vi "SFOAE-Dispose Of Datafile.vi"(0 "Notes":string, 1 "Expt State in":T2, 7 "DataProc":T1, 11 "error in (no error)":errorcluster, 12 "abort":bool) -> (3 "Expt State out":T2, 4 "DataPath":path, 15 "error out":errorcluster)   [LabVIEW 2020]
uses:
  CFTS Main Panel SubVIs/CFTS-Experiment State.ctl
  Typedefs/SFOAE-Data Processing.ctl
  CFTS Main Panel SubVIs/CFTS-Data Type Enum.ctl
  epl-vi-lib/Utility VIs/Math VIs/LinSpace (x0-dx-npts).vi
  epl-vi-lib/Utility VIs/Math VIs/Linear to dB (2D).vi
  <vilib>/regexp/Match Regular Expression.xnode
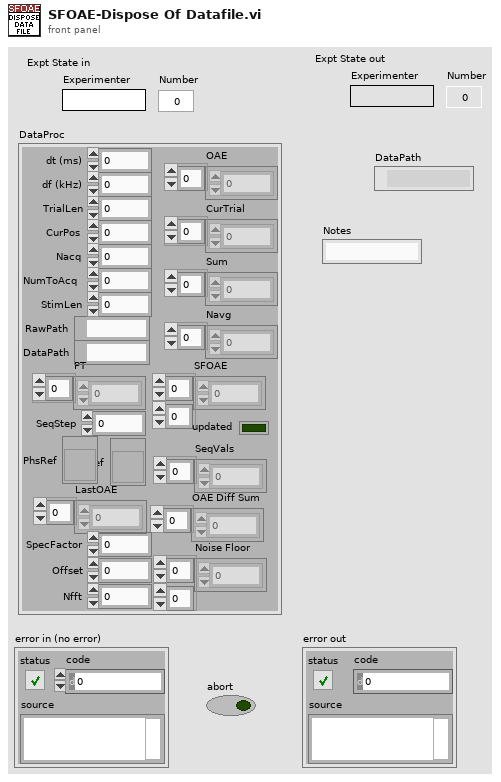
[diagram p1: front panel]
types:
  T1 = typedef "SFOAE-Data Processing.ctl" = cluster{"dt (ms)":dbl, "TrialLen":i32, "PT":cdb[], "CurPos":i32, "Sum":dbl[], "Navg":dbl[], "Nacq":i32, "RawPath":path, "DataPath":path, "NumToAcq":i32, "OAE":dbl[], "CurTrial":dbl[], "StimLen":i32, "SFOAE":cdb[][], "SeqStep":i32, "updated":bool, "SeqVals":dbl[], "df (kHz)":dbl, "MagRef":refnum<vi>, "LastOAE":dbl[], "OAE Diff Sum":dbl[], "Noise Floor":cdb[][], "SpecFactor":dbl, "Offset":i32, "Nfft":i32, "PhsRef":refnum<vi>}
  T2 = typedef "CFTS-Experiment State.ctl" = cluster{"Experimenter":string, "Number":u32, "Right":string, "Left":string, "Data Folder":path, "State File":path, "Version Info":string, "End Exposure Time":dbl, "Exposure Duration":string, "Run #":cluster{"CAP":i16, "ABR":i16, "DP":i16, "VsEP":i16, "MeasSeq":i16, "SubSeq":i16, "SFOAE":i16}}
  T3 = typedef "CFTS-Data Type Enum.ctl" = enum16{"CAP", "ABR", "DP", "VsEP", "MeasSeq", "SFOAE"}
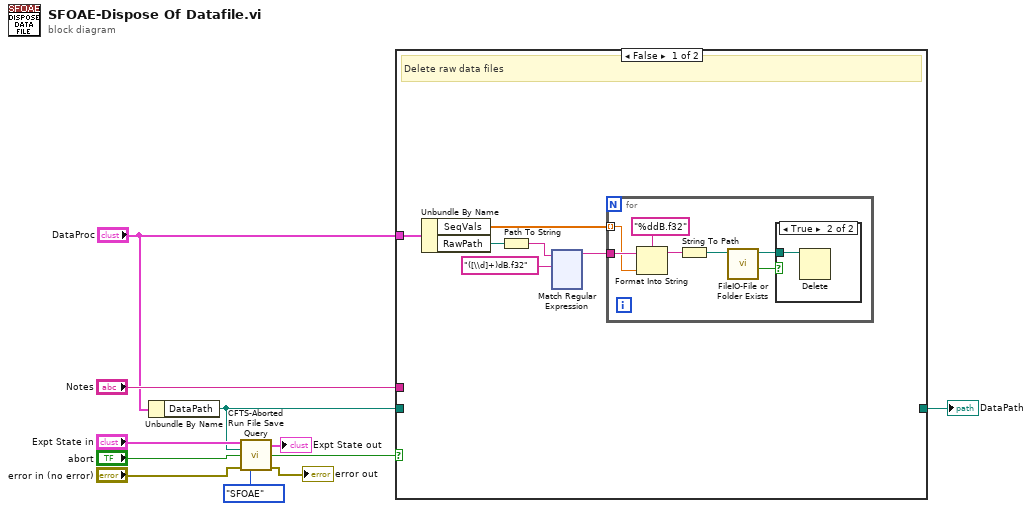
[diagram p0: block diagram]
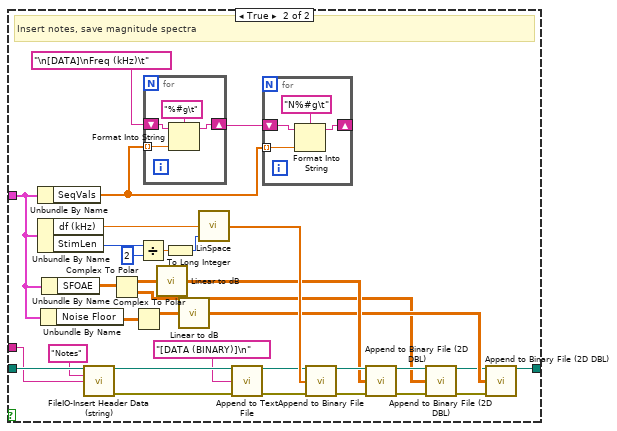
[diagram p3: hidden frame]
diagram:
  n1 = Unbundle By Name("DataProc") -> ("DataPath"=w2:path)
  n2 = call "CFTS-Aborted Run File Save Query.vi"("Expt State"="Expt State in", "Path"=w2, "Aborted"="abort", "error in (no error)"="error in (no error)", "Data Type"=CFTS-Data_Type_Enum."SFOAE") -> ("Expt State out"=→"Expt State out":T2, "File saved?"=w5:bool, "error out"=→"error out":errorcluster)  [unwired: 8 in]
  n3 = case shown="False" w5 {
    tunnel: "Notes" -> [_ w166]
    tunnel: "DataProc" -> [w17 w162]
    tunnel: w2 -> [_ w168]
    tunnel: [_ w143] -> w1
    frame False {
      # "Delete raw data files"
      n4 = Unbundle By Name(w17) -> ("SeqVals"=w16:dbl[], "RawPath"=w13:path)
      n5 = Path To String(path=w13) -> (string=w14:string)
      n6 = xnode "Match Regular Expression"("input string"=w14, "regular expression"="([\\d]+)dB.f32" ("regular expression (\"\")")) -> ("before match"=w12:string)  [unwired: 4 in, 4 out]
      n7 = for {
        tunnel: w16 -> [w134] mode=indexing
        tunnel: w12 -> [w135]
        n8 = Format Into String(format string="%ddB.f32", initial string=w135, w134) -> (resulting string=w132:string)  [unwired: 1 in, 1 out]
        n9 = String To Path(string=w132) -> (path=w131:path)
        n10 = call "FileIO-File or Folder Exists.vi"("path"=w131) -> ("Exists?"=w130:bool, "dup path"=w129:path)  [unwired: 7 in, 2 out]
        n11 = case shown="True" w130 {
          tunnel: w129 -> [_ w136]
          frame False {
          }
          frame True {
            n12 = Delete(path (use dialog)=w136) -> ()  [unwired: 4 in, 3 out]
          }
        }
      }
    }
    frame True {
      # "Insert notes, save magnitude spectra"
      n13 = Unbundle By Name(w162) -> ("SeqVals"=w163:dbl[])
      n14 = Unbundle By Name(w162) -> ("df (kHz)"=w155:dbl, "StimLen"=w157:i32)
      n15 = Unbundle By Name(w162) -> ("Noise Floor"=w158:cdb[][])
      n16 = Unbundle By Name(w162) -> ("SFOAE"=w161:cdb[][])
      n17 = call "FileIO-Insert Header Data (string).vi"("path"=w168, "Field"="Notes", "Data"=w166) -> ("path out"=w148:path, "error out"=w149:errorcluster)  [unwired: 11 in]
      n18 = Complex To Polar(r * e^(i*theta)=w161) -> (r=w160:dbl[][], theta=w137:dbl[][])
      n19 = Complex To Polar(r * e^(i*theta)=w158) -> (r=w159:dbl[][])  [unwired: 1 out]
      n20 = Divide(x=w157, y=2) -> (x/y=w154:dbl)
      n21 = for {
        tunnel: w163 -> [w176] mode=indexing
        shift-right: [w174] -> w164
        shift-left: "\n[DATA]\nFreq (kHz)\t" -> [w175]
        n22 = Format Into String(format string="%#g\t", initial string=w175, w176) -> (resulting string=w174:string)  [unwired: 1 in, 1 out]
      }
      n23 = call-poly "Linear to dB.vi"("linear"=w160) -> ("dB"=w150:dbl[][])
      n24 = To Long Integer(number=w154) -> (32bit integer=w153:i32)
      n25 = call-poly "Linear to dB.vi"("linear"=w159) -> ("dB"=w142:dbl[][])
      n26 = call-poly "LinSpace.vi"("npts"=w153, "dx"=w155) -> ("Array"=w152:dbl[])  [unwired: 2 in, 1 out]
      n27 = call "Append to Text File.vi"("file path"=w148, "text"="[DATA (BINARY)]\n", "error in (no error)"=w149) -> ("file path out"=w145:path, "error out"=w146:errorcluster)  [unwired: 11 in]
      n28 = for {
        tunnel: w163 -> [w172] mode=indexing
        shift-right: [w170] -> _
        shift-left: w164 -> [w171]
        n29 = Format Into String(format string="N%#g\t", initial string=w171, w172) -> (resulting string=w170:string)  [unwired: 1 in, 1 out]
      }
      n30 = call "Append to Binary File.vi"("file path"=w145, "data"=w152, "error in (no error)"=w146) -> ("file path out"=w151:path, "error out"=w144:errorcluster)  [unwired: 11 in]
      n31 = call "Append to Binary File (2D DBL).vi"("file path"=w151, "data"=w150, "error in (no error)"=w144) -> ("file path out"=w138:path, "error out"=w141:errorcluster)  [unwired: 11 in]
      n32 = call "Append to Binary File (2D DBL).vi"("file path"=w138, "data"=w137, "error in (no error)"=w141) -> ("file path out"=w139:path, "error out"=w140:errorcluster)  [unwired: 11 in]
      n33 = call "Append to Binary File (2D DBL).vi"("file path"=w139, "data"=w142, "error in (no error)"=w140) -> ("file path out"=w143:path)  [unwired: 11 in, 1 out]
    }
  }
  "DataPath" <- w1
